vi "Make Node Name Unique.vi"(6 "T: Ignore Repeat Root":bool, 9 "New Node Name":string, 10 "Parent Path":string, 11 "Tree Map In":T1) -> (1 "T: key not found?":bool, 2 "Node Path":string)   [LabVIEW 2021, in "Tree Map.lvlib"]
doc: "<b>Author:</b> Piotr Kruczkowski <PrimaryKey>\n<b>License:</b> NewBSD\n\nCopyright (c) 2019, National Instruments\nAll rights reserved.\n\nRedistribution and use in source and binary forms, with or without\nmodification, are permitted provided that the following conditions are met:\n1. Redistributions of source code must retain the above copyright\n notice, this list of conditions and the following disclaimer.\n2. Redistributions in binary form must reproduce the above copyright\n notice, this list of conditions and the following disclaimer in the\n documentation and/or other materials provided with the distribution.\n3. Neither the name of National Instruments nor the\n names of its contributors may be used to endorse or promote products\n derived from this software without specific prior written permission.\n\nTHIS SOFTWARE IS PROVIDED BY National Instruments ''AS IS'' AND ANY\nEXPRESS OR IMPLIED WARRANTIES, INCLUDING, BUT NOT LIMITED TO, THE IMPLIED\nWARRANTIES OF MERCHANTABILITY AND FITNESS FOR A PARTICULAR PURPOSE ARE\nDISCLAIMED. IN NO EVENT SHALL National Instruments BE LIABLE FOR ANY\nDIRECT, INDIRECT, INCIDENTAL, SPECIAL, EXEMPLARY, OR CONSEQUENTIAL DAMAGES\n(INCLUDING, BUT NOT LIMITED TO, PROCUREMENT OF SUBSTITUTE GOODS OR SERVICES;\nLOSS OF USE, DATA, OR PROFITS; OR BUSINESS INTERRUPTION) HOWEVER CAUSED AND\nON ANY THEORY OF LIABILITY, WHETHER IN CONTRACT, STRICT LIABILITY, OR TORT\n(INCLUDING NEGLIGENCE OR OTHERWISE) ARISING IN ANY WAY OUT OF THE USE OF THIS\nSOFTWARE, EVEN IF ADVISED OF THE POSSIBILITY OF SUCH DAMAGE."
uses:
  <vilib>/National Instruments/Tree Map/Tree Map.lvlib
  <vilib>/National Instruments/Tree Map/Tree Map Data.ctl
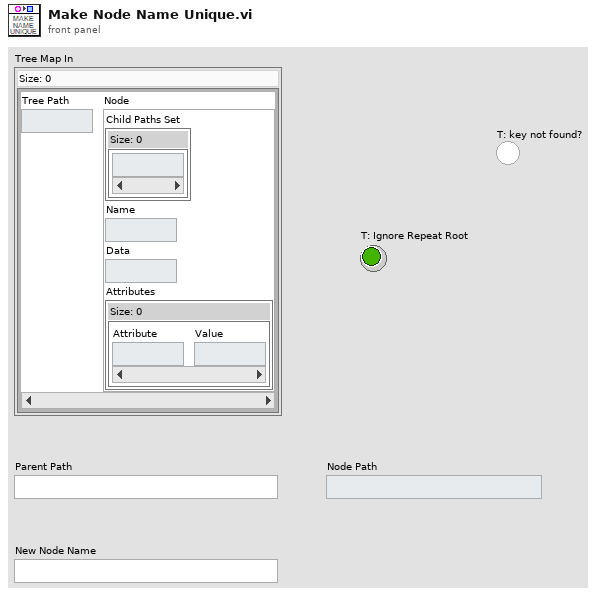
[diagram p1: front panel]
types:
  T1 = typedef "Tree Map.lvlib/Tree Map Data.ctl" = map{string, cluster{"Child Paths Set":set{string}, "Name":string, "Data":string, "Attributes":map{string, string}}}
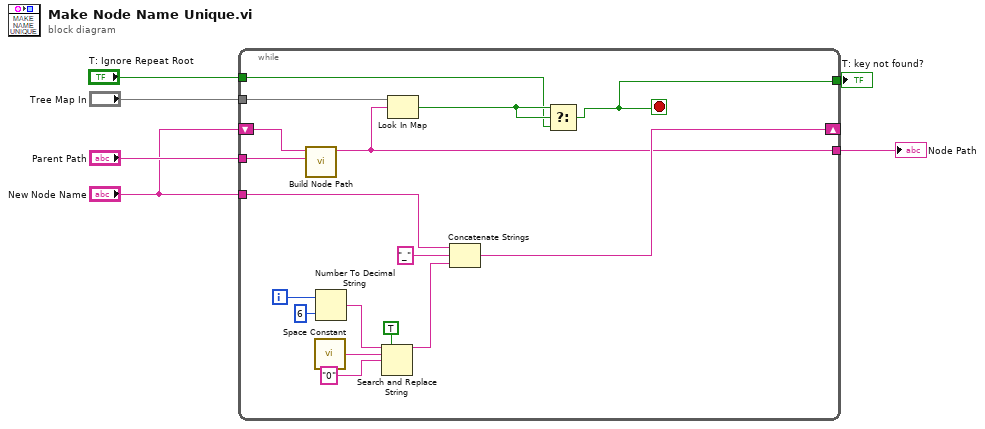
[diagram p0: block diagram]
diagram:
  n1 = while {
    tunnel: "Tree Map In" -> [w23]
    tunnel: "Parent Path" -> [w22]
    shift-right: [w19] -> _
    shift-left: "New Node Name" -> [w21]
    tunnel: [w18] -> w6
    tunnel: "New Node Name" -> [w17]
    tunnel: [w8] -> w2
    tunnel: "T: Ignore Repeat Root" -> [w7]
    i -> [w14]
    stop <- w8 stop-if-true
    n2 = call <vilib>:"Build Node Path.vi"("Parent Path"=w22, "Node Name"=w21) -> ("Node Path"=w18:string)  [unwired: 9 in]
    n3 = call <vilib>:"Space Constant.vi"() -> ("String"=w12:string)
    n4 = Number To Decimal String(number=w14, width (-)=i16 6) -> (decimal integer string=w13:string)
    n5 = Search and Replace String(replace all?=TRUE ("replace all? (F)"), input string=w13, search string=w12, replace string="0" ("replace string (\"\")")) -> (result string=w10:string)  [unwired: 4 in, 3 out]
    n6 = Look In Map(map=w23, key=w18) -> (key not found?=w9:bool)  [unwired: 1 in, 1 out]
    n7 = Concatenate Strings(w17, "_" ("string"), w10) -> (w19:string)
    n8 = Select(t=w9, s=w9, f=w7) -> (s? t:f=w8:bool)
  }
  "Node Path" <- w6
  "T: key not found?" <- w2
